vi "ColorChange.vi"(8 "error in (no error)":errorcluster, 9 "Image Dst":T1, 10 "Image Src":T1, 11 "Enum":enum16{"Blue", "Red", "Purple", "Test"}(ring)) -> (0 "error out":errorcluster, 3 "Image Dst Out":T1)   [LabVIEW 2011]
uses:
  <vilib>/vision/Image Controls.llb/IMAQ Image.ctl
  <vilib>/vision/NI_Vision_Development_Module.lvlib
panel:
  in  "?":enum32{"Blue", "Red", "Purple", "Test"}(tab)
  in  "Margins 3":cluster{"Hue":i32, "Sat":i32, "Lum":i32}={"Hue"=12, "Sat"=0, "Lum"=0}
  in  "Hue 3":i32(knob)=160 scale=0.0..255.0
  in  "Saturation 3":i32=120
  in  "Luminance 3":i32=20
  in  "Margins 2":cluster{"Hue":i32, "Sat":i32, "Lum":i32}={"Hue"=20, "Sat"=0, "Lum"=0}
  in  "Hue 2":i32(knob)=250 scale=0.0..255.0
  in  "Saturation 2":i32=30
  in  "Luminance 2":i32=50
  in  "Margins 4":cluster{"Hue":i32, "Sat":i32, "Lum":i32}={"Hue"=22, "Sat"=10, "Lum"=0}
  in  "Hue 4":i32(knob)=211 scale=0.0..255.0
  in  "Saturation 4":i32=75
  in  "Luminance 4":i32=60
  in  "Margins 5":cluster{"Hue":i32, "Sat":i32, "Lum":i32}={"Hue"=15, "Sat"=15, "Lum"=7} {"Sat" scale=0.0..40.0; "Lum" scale=0.0..40.0; "Hue" scale=0.0..40.0}
  in  "Hue 5":i32(knob)=170 scale=0.0..255.0
  in  "Saturation 5":i32=100
  in  "Luminance 5":i32=19
  # "This VI filters the incoming\nPicture by HSL color.\nOutput produced is a binary\nimage of pixels within threshold."
  # "Hue3: 191\nSat3: 100\nLum3: 50\nHueMarg3: 40\nSat Marg3: 0\nLum Marg3: 25"
  # "Hue2: 255\nSat2: 0\nLum2: 100\nHue Marg: 28\nSat Marg2: 0\nLum Marg2: 0"
  # "ALT\nHue  210\nSat 115\nLum 60\nMargin:\nHue 22\nSat 0\nLum 0"
  # "Hue  224\nSat 130\nLum 55\nMargin:\nHue 40\nSat 0\nLum 0"
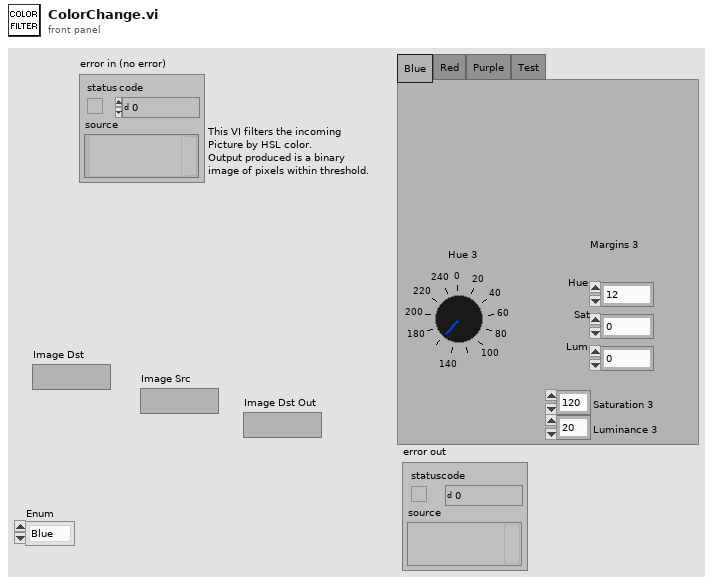
[diagram p1: front panel]
types:
  T1 = typedef "IMAQ Image.ctl" = refnum<image>
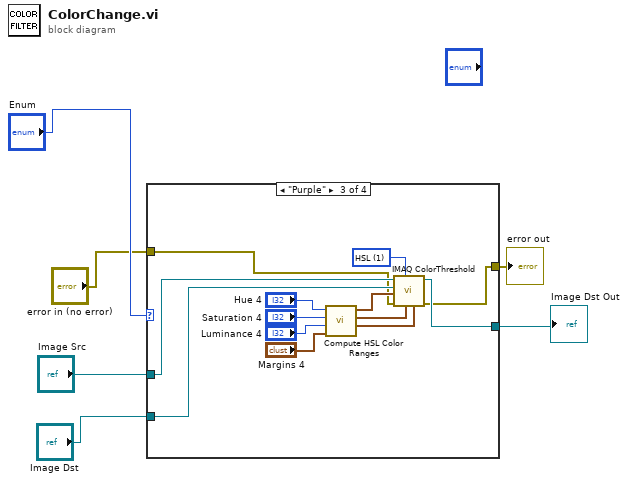
[diagram p0: block diagram]
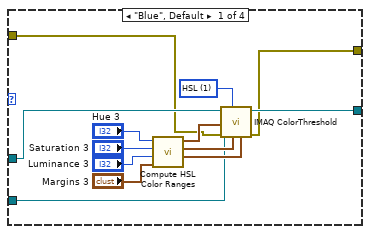
[diagram p2: hidden frame]
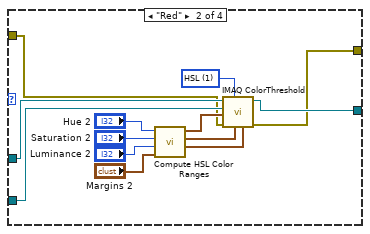
[diagram p3: hidden frame]
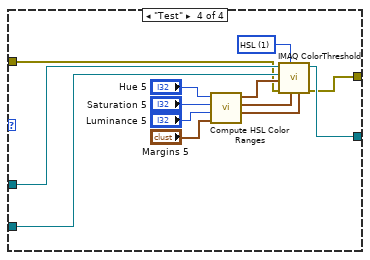
[diagram p4: hidden frame]
diagram:
  n1 = case shown="\"Purple\"" "Enum" {
    tunnel: "Image Src" -> [w11 w24 w35 w50]
    tunnel: "Image Dst" -> [w10 w23 w36 w49]
    tunnel: [w9 w22 w37 w48] -> w4
    tunnel: "error in (no error)" -> [w8 w21 w34 w47]
    tunnel: [w7 w20 w33 w46] -> w1
    frame "Blue", Default {
      w19 = u16 1 items=["RGB", "HSL", "HSV", "HSI"] ("Color Mode")
      n2 = call "Compute HSL Color Ranges.vi"("Margins"="Margins 3", "Luminance"="Luminance 3", "Saturation"="Saturation 3", "Hue"="Hue 3") -> ("Lum Range"=w16:cluster{i32, i32}, "Sat Range"=w17:cluster{i32, i32}, "Hue Range"=w18:cluster{i32, i32})  [unwired: 5 in]
      n3 = call "IMAQ ColorThreshold"("Blue or Luma or Val or Inten Range"=w16, "Green or Sat Range"=w17, "Color Mode"=w19, "error in (no error)"=w8, "Red or Hue Range"=w18, "Image Dst"=w10, "Image Src"=w11) -> ("error out"=w7:errorcluster, "Image Dst Out"=w9:T1)  [unwired: 3 in]
    }
    frame "Red" {
      w32 = u16 1 items=["RGB", "HSL", "HSV", "HSI"] ("Color Mode")
      n4 = call "Compute HSL Color Ranges.vi"("Margins"="Margins 2", "Luminance"="Luminance 2", "Saturation"="Saturation 2", "Hue"="Hue 2") -> ("Lum Range"=w29:cluster{i32, i32}, "Sat Range"=w30:cluster{i32, i32}, "Hue Range"=w31:cluster{i32, i32})  [unwired: 5 in]
      n5 = call "IMAQ ColorThreshold"("Blue or Luma or Val or Inten Range"=w29, "Green or Sat Range"=w30, "Color Mode"=w32, "error in (no error)"=w21, "Red or Hue Range"=w31, "Image Dst"=w23, "Image Src"=w24) -> ("error out"=w20:errorcluster, "Image Dst Out"=w22:T1)  [unwired: 3 in]
    }
    frame "Purple" {
      w38 = u16 1 items=["RGB", "HSL", "HSV", "HSI"] ("Color Mode")
      n6 = call "Compute HSL Color Ranges.vi"("Margins"="Margins 4", "Luminance"="Luminance 4", "Saturation"="Saturation 4", "Hue"="Hue 4") -> ("Lum Range"=w41:cluster{i32, i32}, "Sat Range"=w40:cluster{i32, i32}, "Hue Range"=w39:cluster{i32, i32})  [unwired: 5 in]
      n7 = call "IMAQ ColorThreshold"("Blue or Luma or Val or Inten Range"=w41, "Green or Sat Range"=w40, "Color Mode"=w38, "error in (no error)"=w34, "Red or Hue Range"=w39, "Image Dst"=w36, "Image Src"=w35) -> ("error out"=w33:errorcluster, "Image Dst Out"=w37:T1)  [unwired: 3 in]
    }
    frame "Test" {
      w51 = u16 1 items=["RGB", "HSL", "HSV", "HSI"] ("Color Mode")
      n8 = call "Compute HSL Color Ranges.vi"("Margins"="Margins 5", "Luminance"="Luminance 5", "Saturation"="Saturation 5", "Hue"="Hue 5") -> ("Lum Range"=w54:cluster{i32, i32}, "Sat Range"=w53:cluster{i32, i32}, "Hue Range"=w52:cluster{i32, i32})  [unwired: 5 in]
      n9 = call "IMAQ ColorThreshold"("Blue or Luma or Val or Inten Range"=w54, "Green or Sat Range"=w53, "Color Mode"=w51, "error in (no error)"=w47, "Red or Hue Range"=w52, "Image Dst"=w49, "Image Src"=w50) -> ("error out"=w46:errorcluster, "Image Dst Out"=w48:T1)  [unwired: 3 in]
    }
  }
  "Image Dst Out" <- w4
  "error out" <- w1
